vi "microStepLoop.vi"(0 "StepsInAramp":i16, 5 "CorrectedIncrement":i16, 7 "ResetUstep":bool, 9 "Clock Trigger":bool) -> (4 "CurrentUstep":i16, 6 "NextUstep":i16, 8 "BotRamp":bool, 10 "MaxPulse":bool, 15 "TopRamp":bool)   [LabVIEW 2016]
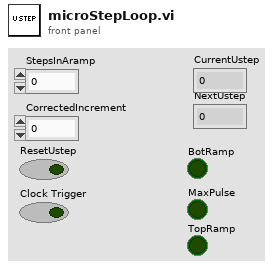
[diagram p1: front panel]
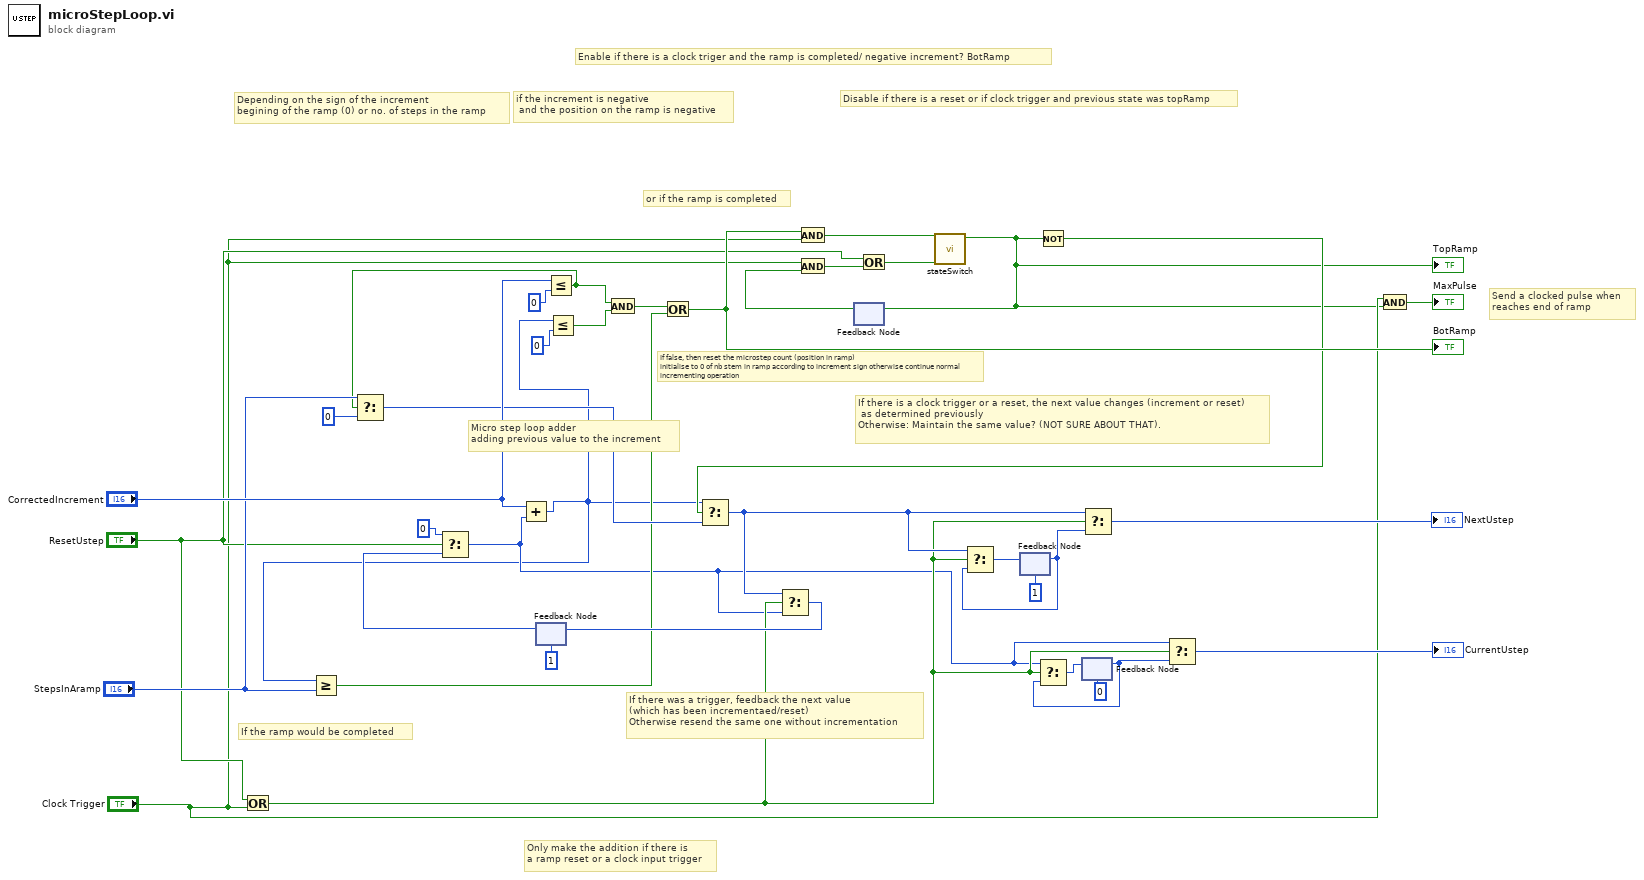
[diagram p0: block diagram]
diagram:
  # "Disable if there is a reset or if clock trigger and previous state was topRamp"
  # "Enable if there is a clock triger and the ramp is completed/ negative increment? BotRamp"
  # "or if the ramp is completed"
  # "If there was a trigger, feedback the next value \n(which has been incrementaed/reset)\nOtherwise resend the same one without incrementation"
  # "If there is a clock trigger or a reset, the next value changes (increment or reset)\n as determined previously\nOtherwise: Maintain the same value? (NOT SURE ABOUT THAT)."
  # "If false, then reset the microstep count (position in ramp)\ninitialise to 0 of nb stem in ramp according to increment sign otherwise continue normal incrementing operation"
  # "Depending on the sign of the increment\nbegining of the ramp (0) or no. of steps in the ramp"
  # "if the increment is negative \n and the position on the ramp is negative"
  # "Only make the addition if there is\na ramp reset or a clock input trigger"
  # "Send a clocked pulse when\nreaches end of ramp"
  # "Micro step loop adder\nadding previous value to the increment"
  # "If the ramp would be completed"
  n1 = Or(x="ResetUstep", y="Clock Trigger") -> (x .or. y?=w12:bool)
  n2 = feedback #1(i16 1) -> (w34:i16)
  n3 = Select(t=i16 0, s="ResetUstep", f=w34) -> (s? t:f=w2:i16)
  n4 = Add(x="CorrectedIncrement", y=w2) -> (x+y=w1:i16)
  n5 = Greater Or Equal?(x=w1, y="StepsInAramp") -> (x >= y?=w17:bool)
  n6 = Less Or Equal?(x="CorrectedIncrement", y=i16 0) -> (x <= y?=w26:bool)
  n7 = Select(t="StepsInAramp", s=w26, f=i16 0) -> (s? t:f=w25:i16)
  n8 = Less Or Equal?(x=w1, y=i16 0) -> (x <= y?=w29:bool)
  n9 = And(x=w26, y=w29) -> (x .and. y?=w18:bool)
  n10 = Or(x=w18, y=w17) -> (x .or. y?=w11:bool)
  "BotRamp" <- w11
  n11 = And(x=w11, y="Clock Trigger") -> (x .and. y?=w10:bool)
  n12 = feedback #2() -> (w3:bool)  [unwired: 1 in]
  n13 = And(x="Clock Trigger", y=w3) -> (x .and. y?=w8:bool)
  n14 = Or(x="ResetUstep", y=w8) -> (x .or. y?=w9:bool)
  n15 = call "stateSwitch.vi"("disable"=w9, "enable"=w10) -> ("state"=w4:bool)  [unwired: 9 in]
  "TopRamp" <- w4
  n16 = feedback-in #2(w4) -> ()
  n17 = feedback #3(i16 1) -> (w22:i16)
  n18 = Not(x=w4) -> (.not. x?=w5:bool)
  n19 = Select(t=w1, s=w5, f=w25) -> (s? t:f=w20:i16)
  n20 = Select(t=w20, s=w12, f=w2) -> (s? t:f=w19:i16)
  n21 = feedback-in #1(w19) -> ()
  n22 = Select(t=w20, s=w12, f=w22) -> (s? t:f=w23:i16)
  n23 = feedback-in #3(w23) -> ()
  n24 = feedback #4(i16 0 ("t")) -> (w15:i16)
  n25 = Select(t=w2, s=w12, f=w15) -> (s? t:f=w16:i16)
  n26 = feedback-in #4(w16) -> ()
  n27 = Select(t=w20, s=w12, f=w22) -> (s? t:f=→"NextUstep":i16)
  n28 = Select(t=w2, s=w12, f=w15) -> (s? t:f=→"CurrentUstep":i16)
  n29 = And(x="Clock Trigger", y=w4) -> (x .and. y?=→"MaxPulse":bool)
